vi "Setup.vi"(8 "Error in":errorcluster, 11 "EVE reference in":refnum<data-value>) -> (0 "error out":errorcluster, 3 "EVE reference out":refnum<data-value>)   [LabVIEW 2013]
uses:
  Class/EVE/EVE.lvclass
  090 - ERRORS/Ctrls/EnumErrors.ctl
  050 - CONFIG/00 - ApplicationConfig/Ctrls/EnumFgvConfigCommand.ctl
  100_PROCESS/SubVis/EnumFgvReferenceProcess.ctl
  100_PROCESS/Class/Process/EnumProcess.ctl
  100_PROCESS/01_MessageHandlerProcess/Class/MessageHandler.lvclass
  100_PROCESS/00_Template/Class/Template.lvclass
  100_PROCESS/Class/Process/Process.lvclass
  090 - ERRORS/Ctrls/enumLogAndView.ctl
  030 - EVENTS/03 - ToMessageHandlerProcess/enumMessageCriticity.ctl
panel:
  # "SETUP"
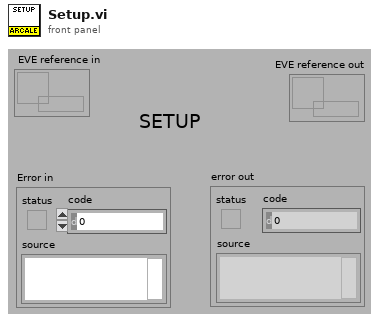
[diagram p1: front panel]
types:
  T1 = typedef "EnumErrors.ctl" = enum16{"VI non trouvé !", "Clé non trouvée", "Timeout", "Le VI tourne déjà", "Erreur de séparateur décimal", "Référence non trouvée"}
  T2 = typedef "EnumFgvConfigCommand.ctl" = enum16{"Load", "Get", "Set", "Save To Disk"}
  T3 = typedef "EnumFgvReferenceProcess.ctl" = enum16{"Init", "Get", "Add Reference", "Close References"}
  T4 = typedef "Process.lvclass/EnumProcess.ctl" = enum16{"Message handler", "Template"}
  T5 = typedef "enumMessageCriticity.ctl" = enum16{"No error", "Info", "Warning", "Error", "Fatal error"}
  T6 = typedef "enumLogAndView.ctl" = enum16{"Log only", "Log and view"}
  T7 = typedef "BenchConfig.ctl" = cluster{"Cfg":string}
  T8 = typedef "paramsExternalProcesses.ctl" = cluster{"Path":path, "Timeout":dbl, "viInitString":string, "State":enum32{"Invalid", "Standard", "Closed", "Hidden", "Minimized", "Maximized"}}
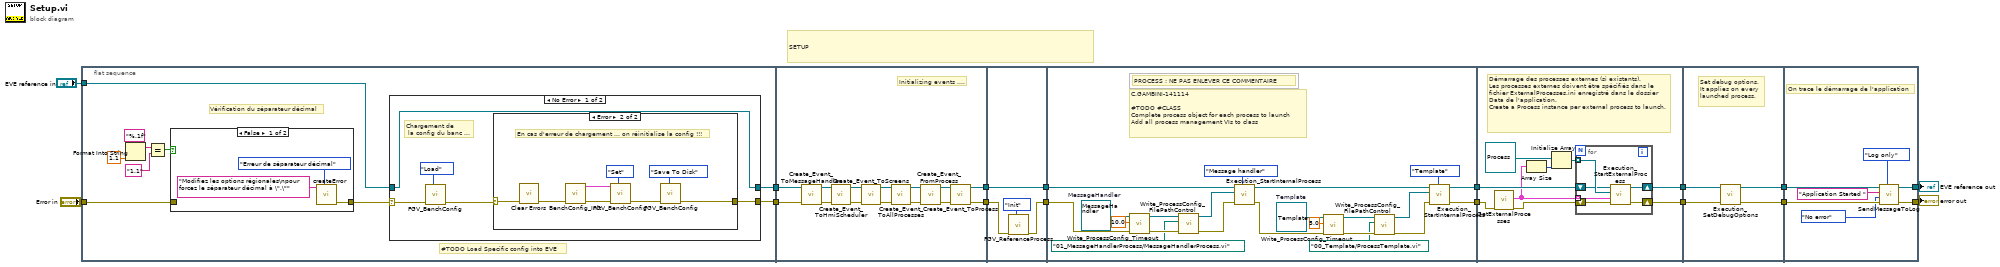
[diagram p0: block diagram]
diagram:
  # "SETUP"
  n1 = flat-sequence {
    tunnel: [w26] -> w14
    tunnel: "Error in" -> [w19]
    tunnel: "EVE reference in" -> [w18]
    tunnel: [w17] -> w1
    tunnel: w14 -> [w60]
    tunnel: [w50] -> w12
    tunnel: [w48] -> w10
    tunnel: w1 -> [w47]
    tunnel: w12 -> [w64]
    tunnel: [w63] -> w11
    tunnel: w10 -> [w61]
    tunnel: [w61] -> w9
    tunnel: w11 -> [w81]
    tunnel: [w65] -> w13
    tunnel: w9 -> [w86]
    tunnel: [w83] -> w8
    tunnel: [w95] -> w6
    tunnel: w13 -> [w93]
    tunnel: [w87] -> w4
    tunnel: w8 -> [w92]
    tunnel: w6 -> [w105]
    tunnel: [w104] -> w5
    tunnel: w4 -> [w103]
    tunnel: [w102] -> w3
    tunnel: [w112] -> w15
    tunnel: w5 -> [w109]
    tunnel: w3 -> [w107]
    tunnel: [w106] -> w2
    frame #0 {
      # "#TODO Load Specific config into EVE"
      # "Vérification du séparateur décimal"
      n2 = Format Into String(format string="%.1f", 1.1) -> (resulting string=w22:string)  [unwired: 2 in, 1 out]
      n3 = Equal?(x=w22, y="1.1") -> (x = y?=w20:bool)
      n4 = case shown="False" w20 {
        tunnel: w19 -> [_ w30]
        tunnel: [w29 w30] -> w25
        frame False {
          n5 = call "createError.vi"("ErrorCode"=EnumErrors."Erreur de séparateur décimal", "message"="Modifiez les options régionales\npour forcez le séparateur décimal à \".\"") -> ("error out"=w29:errorcluster)  [unwired: 9 in]
        }
        frame True {
        }
      }
      n6 = case shown="No Error" w25 {
        selector: w25 -> [w35 w46]
        tunnel: [w32 w46] -> w26
        tunnel: w18 -> [w31 w45]
        tunnel: [w31 w45] -> w17
        frame No Error {
          # "Chargement de\n la config du banc ..."
          n7 = call "FGV_BenchConfig.vi"("Command"=EnumFgvConfigCommand."Load", "error in (no error)"=w35) -> ("error out"=w33:errorcluster)  [unwired: 8 in, 1 out]
          n8 = case shown="Error" w33 {
            selector: w33 -> [w36 w39]
            tunnel: [w36 w38] -> w32
            frame No Error {
            }
            frame Error {
              # "En cas d'erreur de chargement ... on réinitialise la config !!!"
              n9 = call <vilib>:"Clear Errors.vi"("error in (no error)"=w39) -> ("error out"=w37:errorcluster)  [unwired: 6 in]
              n10 = call "BenchConfig_Init.vi"("error in (no error)"=w37) -> ("error out"=w42:errorcluster, "BenchConfig"=w43:T7)  [unwired: 9 in]
              n11 = call "FGV_BenchConfig.vi"("Command"=EnumFgvConfigCommand."Set", "error in (no error)"=w42, "BenchConfigIn"=w43) -> ("error out"=w40:errorcluster)  [unwired: 7 in, 1 out]
              n12 = call "FGV_BenchConfig.vi"("Command"=EnumFgvConfigCommand."Save To Disk", "error in (no error)"=w40) -> ("error out"=w38:errorcluster)  [unwired: 8 in, 1 out]
            }
          }
        }
        frame Error {
        }
      }
    }
    frame #1 {
      # "Initializing events ...."
      n13 = call "Create_Event_ToMessageHandler.vi"("Error in"=w60, "EVE reference in"=w47) -> ("Error out"=w59:errorcluster, "EVE reference out"=w58:refnum<data-value>)  [unwired: 8 in]
      n14 = call "Create_Event_ToHmiScheduler.vi"("error in (no error)"=w59, "EVE reference in"=w58) -> ("error out"=w57:errorcluster, "EVE reference out"=w56:refnum<data-value>)  [unwired: 8 in]
      n15 = call "Create_Event_ToScreens.vi"("error in (no error)"=w57, "EVE reference in"=w56) -> ("error out"=w54:errorcluster, "EVE reference out"=w55:refnum<data-value>)  [unwired: 8 in]
      n16 = call "Create_Event_ToAllProcesses.vi"("error in (no error)"=w54, "EVE reference in"=w55) -> ("error out"=w53:errorcluster, "EVE reference out"=w52:refnum<data-value>)  [unwired: 8 in]
      n17 = call "Create_Event_FromProcess.vi"("error in (no error)"=w53, "EVE reference in"=w52) -> ("Error out"=w51:errorcluster, "EVE reference out"=w49:refnum<data-value>)  [unwired: 8 in]
      n18 = call "Create_Event_ToProcess.vi"("error in (no error)"=w51, "EVE reference in"=w49) -> ("error out"=w50:errorcluster, "EVE reference out"=w48:refnum<data-value>)  [unwired: 8 in]
    }
    frame #2 {
      n19 = call "FGV_ReferenceProcess.vi"("Commande"=EnumFgvReferenceProcess."Init", "error in (no error)"=w64) -> ("error out"=w63:errorcluster)  [unwired: 8 in, 1 out]
    }
    frame #3 {
      w71 = refnum<class "Template.lvclass"> refnum  # Template
      w77 = refnum<class "MessageHandler.lvclass"> refnum  # MessageHandler
      # "C.GAMBINI-141114\n\n#TODO #CLASS\nComplete process object for each process to launch\nAdd all process management VIs to class"
      # "PROCESS : NE PAS ENLEVER CE COMMENTAIRE"
      n20 = call-dynamic "Write_ProcessConfig_Timeout.vi"("error in (no error)"=w81, "Timeout (s)"=10.0 ("Timeout"), "Process in"=w77) -> ("error out"=w74:errorcluster, "Process out"=w76:refnum<class "MessageHandler.lvclass">)  [unwired: 7 in]
      n21 = call-dynamic "Write_ProcessConfig_FilePathControl.vi"("error in (no error)"=w74, "File Path Control"=path "01_MessageHandlerProcess/MessageHandlerProcess.vi", "Process in"=w76) -> ("error out"=w73:errorcluster, "Process out"=w75:refnum<class "MessageHandler.lvclass">)  [unwired: 7 in]
      n22 = call-dynamic "Execution_StartInternalProcess.vi"("InternalProcess"=EnumProcess."Message handler" ("Process"), "error in (no error)"=w73, "Process in"=w75, "EVE reference in"=w86) -> ("error out"=w78:errorcluster, "EVE reference out"=w84:refnum<data-value>)  [unwired: 6 in]
      n23 = call-dynamic "Write_ProcessConfig_Timeout.vi"("error in (no error)"=w78, "Timeout (s)"=5.0 ("Timeout"), "Process in"=w71) -> ("error out"=w68:errorcluster, "Process out"=w70:refnum<class "Template.lvclass">)  [unwired: 7 in]
      n24 = call-dynamic "Write_ProcessConfig_FilePathControl.vi"("error in (no error)"=w68, "File Path Control"=path "00_Template/ProcessTemplate.vi", "Process in"=w70) -> ("error out"=w67:errorcluster, "Process out"=w69:refnum<class "Template.lvclass">)  [unwired: 7 in]
      n25 = call-dynamic "Execution_StartInternalProcess.vi"("InternalProcess"=EnumProcess."Template" ("Process"), "error in (no error)"=w67, "Process in"=w69, "EVE reference in"=w84) -> ("error out"=w65:errorcluster, "EVE reference out"=w83:refnum<data-value>)  [unwired: 6 in]
    }
    frame #4 {
      # "Démarrage des processes externes (si existants).\nLes processes externes doivent être spécifiés dans le fichier ExternalProcesses.ini enregistré dans le dossier Data de l'application. \nCreate a Process instance per external process to launch."
      n26 = call "GetExternalProcesses.vi"("Error In"=w93) -> ("Error Out"=w94:errorcluster, "ExternalProcesses"=w89:T8[])  [unwired: 9 in]
      n27 = Array Size(array=w89) -> (size(s)=w91:i32)
      n28 = Initialize Array(refnum<class "Process.lvclass"> refnum ("Process.lvclass"), w91) -> (w88:refnum<class "Process.lvclass">[])
      n29 = for {
        shift-right: [w100] -> w95
        shift-left: w94 -> [w101]
        tunnel: w89 -> [w97] mode=indexing
        shift-right: [w99] -> w87
        shift-left: w92 -> [w96]
        tunnel: w88 -> [w98] mode=indexing
        n30 = call-dynamic "Execution_StartExternalProcess.vi"("error in (no error)"=w101, "ProcessConfig"=w97, "Process in"=w98, "EVE reference in"=w96) -> ("error out"=w100:errorcluster, "EVE reference out"=w99:refnum<data-value>)  [unwired: 6 in]
      }
    }
    frame #5 {
      # "Set debug options.\nIt applies on every\nlaunched process."
      n31 = call "Execution_SetDebugOptions.vi"("error in"=w105, "EVE reference in"=w103) -> ("error out"=w104:errorcluster, "EVE reference out"=w102:refnum<data-value>)  [unwired: 8 in]
    }
    frame #6 {
      # "On trace le démarrage de l'application"
      n32 = call "SendMessageToLog.vi"("Log and view ?"=enumLogAndView."Log only", "error in (no error)"=w109, "Criticity"=enumMessageCriticity."No error", "Message"="Application Started ", "EVE reference in"=w107) -> ("error out"=w112:errorcluster, "EVE reference out"=w106:refnum<data-value>)  [unwired: 5 in]
    }
  }
  "error out" <- w15
  "EVE reference out" <- w2
